vi "LCM_player.vi"() -> ()   [LabVIEW 2015]
uses:
  <vilib>/Utility/file.llb/Write To Spreadsheet File (DBL).vi
  G_LCM.vi
panel:
  out "size(s)":i32
  out "LCM error":errorcluster
  in  "long format":bool
  out "UDP Comm. Error 2":errorcluster
  out "Receive Buffer Size":u32
  out "recv data":string
  out "Array":string[](array[string])
  out "time":dbl
  out "log time":string
  in  "time-to-live":u16
  out "LCM":T1
  out "Wait for next data recv [sec]":dbl
  out "File Path":path
  in  "배속(0.1~10)":dbl=0.2 min=0.01 max=10.0 step=0.01
  out "t_old":i64
  out "idxtime":i64[](array[numeric])
  in  "Sequence Index Slider":i32(slide) scale=0.0..1387934.0
  out "idxsize":i32[](array[numeric])
  in  "Play/Pause":bool
  out "channel":string
  out "header":T2 {"magic" format="%08x"}
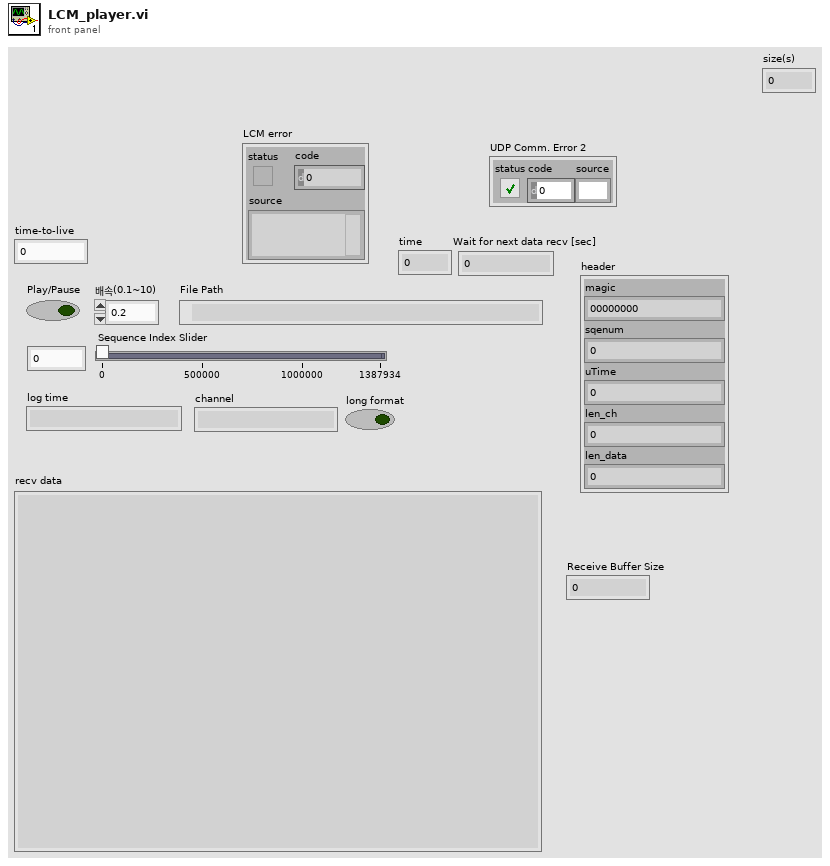
[diagram p1: front panel]
types:
  T1 = cluster{"connection ID":refnum<k16>, "net address":u32, "port":u16}
  T2 = cluster{"magic":i32, "sqenum":i64, "uTime":i64, "len_ch":i32, "len_data":i32}
  T3 = enum8{"Enabled", "Disabled", "Disabled and Grayed Out"}
  T4 = cluster{"magic":u32, "msg_seqno":u32, "msg_size":u32, "fragment_offset":u32, "fragment_no":u16, "fragments_in_msg":u16}
  T5 = cluster{"hash":i64, "sys time":i64, "time":dbl, "yaw_rate":dbl, "mdps torque":dbl, "mdps str_ang":dbl, "VS_CAN":dbl, "lat_accel":dbl, "mcp":dbl, "accel pedal value":dbl, "tps":dbl, "odometer":dbl, "battery voltage":dbl, "WHL_SPD_RR":dbl, "WHL_SPD_RL":dbl, "WHL_SPD_FR":dbl, "WHL_SPD_FL":dbl}
  T6 = cluster{"hash":dbl, "sys time":dbl, "time":dbl, "yaw_rate":dbl, "mdps torque":dbl, "mdps str_ang":dbl, "VS_CAN":dbl, "lat_accel":dbl, "mcp":dbl, "accel pedal value":dbl, "tps":dbl, "odometer":dbl, "battery voltage":dbl, "WHL_SPD_RR":dbl, "WHL_SPD_RL":dbl, "WHL_SPD_FR":dbl, "WHL_SPD_FL":dbl}
  T7 = cluster{"hash":i64, "sys time":i64, "time":dbl, "x":dbl, "y":dbl, "h":dbl, "numSV":i32, "postype":i32, "lag":i32, "hordev":dbl, "lat":dbl, "lon":dbl, "hgt":dbl, "map_idx":i32}
  T8 = cluster{"hash":dbl, "sys time":dbl, "time":dbl, "x":dbl, "y":dbl, "h":dbl, "numSV":dbl, "postype":dbl, "lag":dbl, "hordev":dbl, "lat":dbl, "lon":dbl, "hgt":dbl, "map_idx":dbl}
  T9 = cluster{"hash":i64, "sys time":i64, "time":dbl, "speed":dbl, "heading":dbl, "lat":dbl, "lon":dbl}
  T10 = cluster{"hash":dbl, "sys time":dbl, "time":dbl, "speed":dbl, "heading":dbl, "lat":dbl, "lon":dbl}
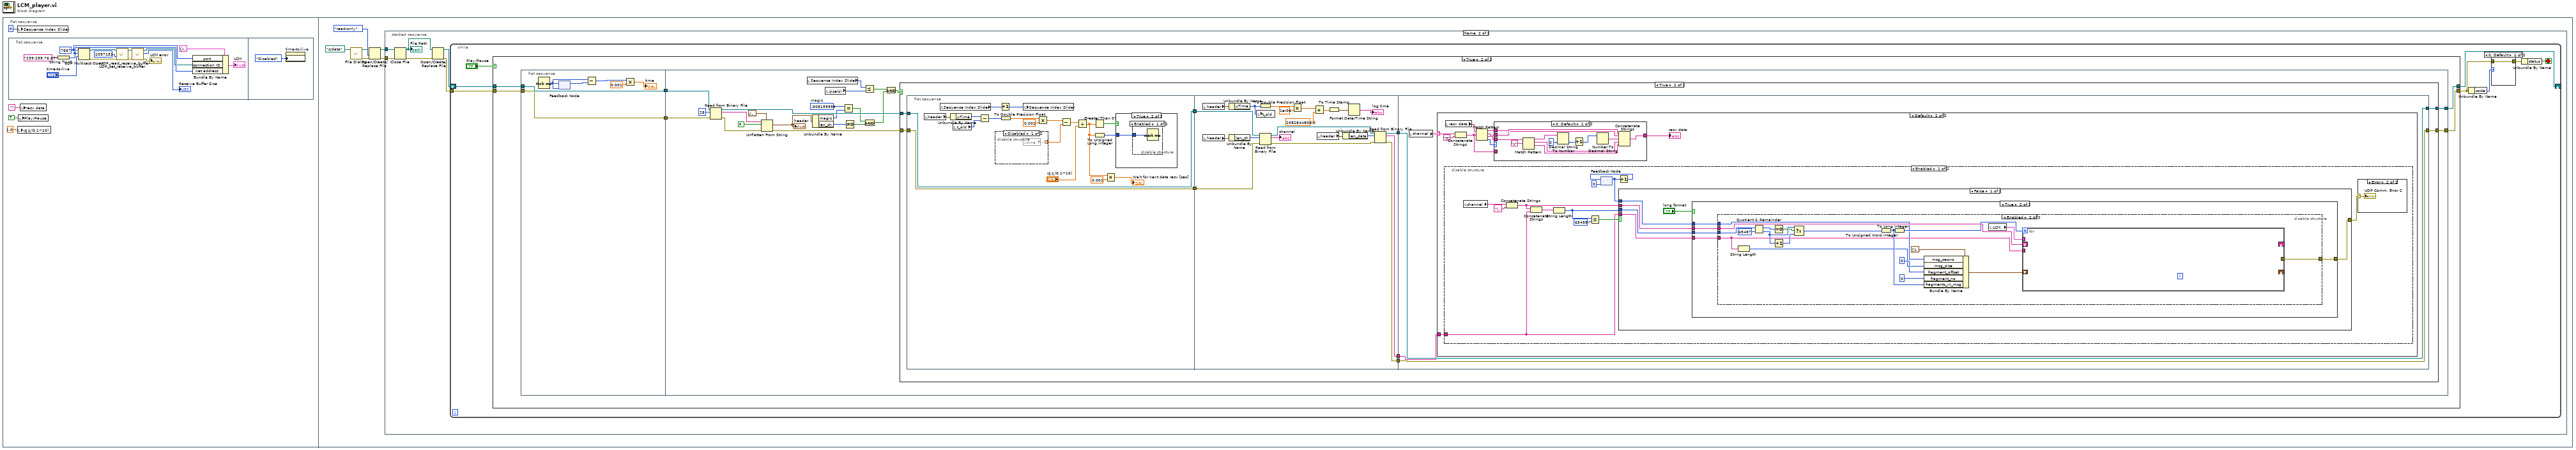
[diagram p0: block diagram]
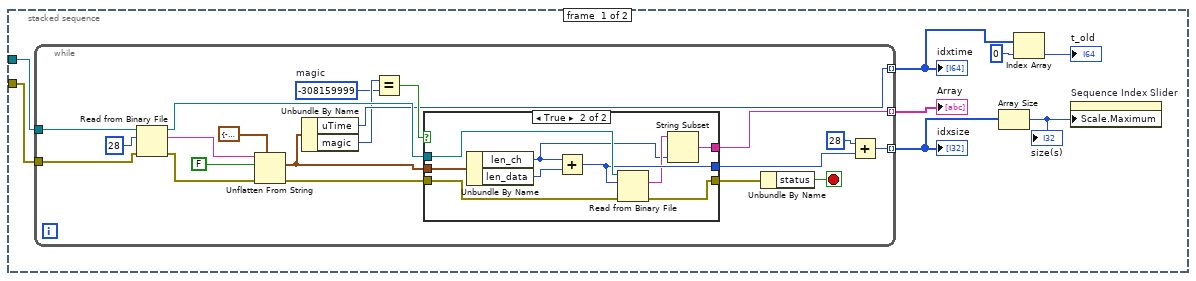
[diagram p2: hidden frame]
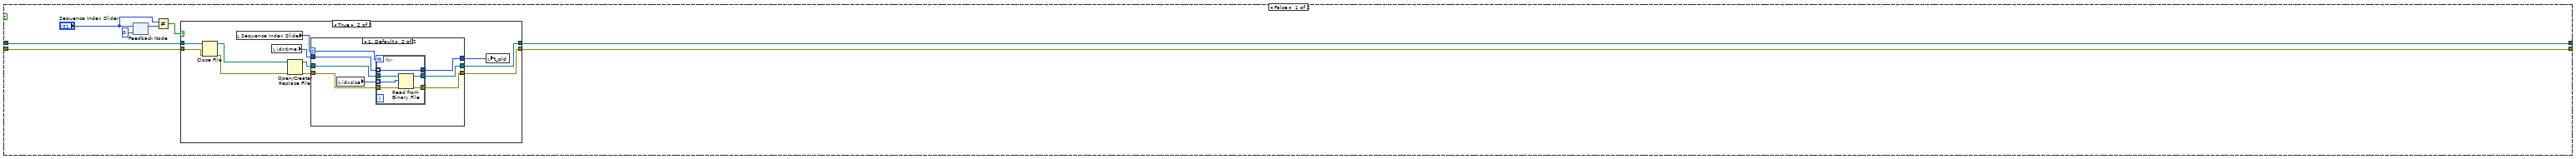
[diagram p5: hidden frame]
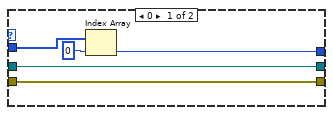
[diagram p7: hidden frame]
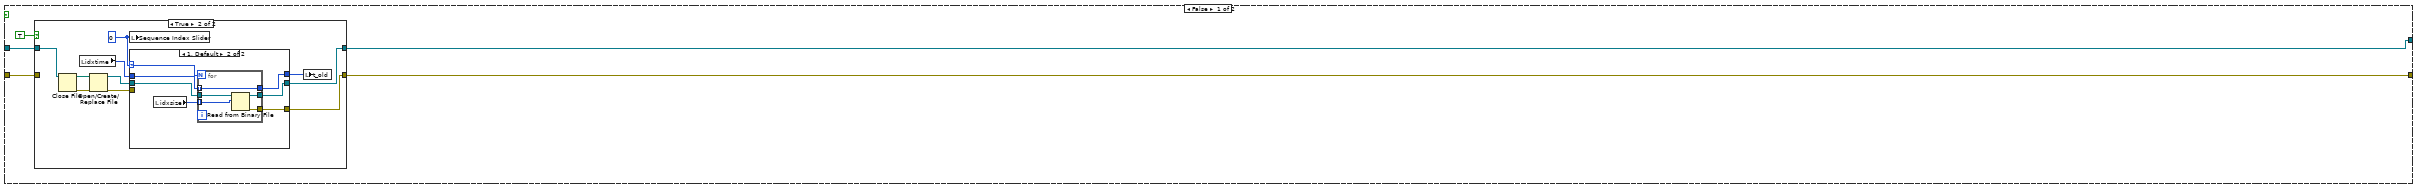
[diagram p8: hidden frame]
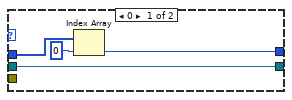
[diagram p10: hidden frame]
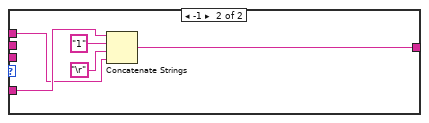
[diagram p15: hidden frame]
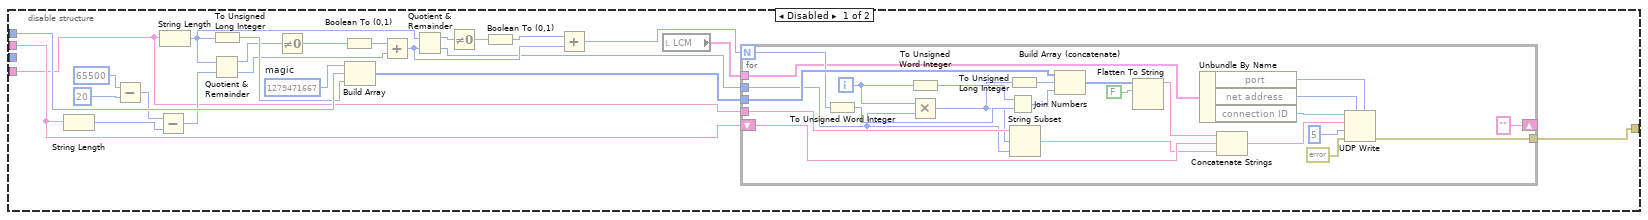
[diagram p17: hidden frame]
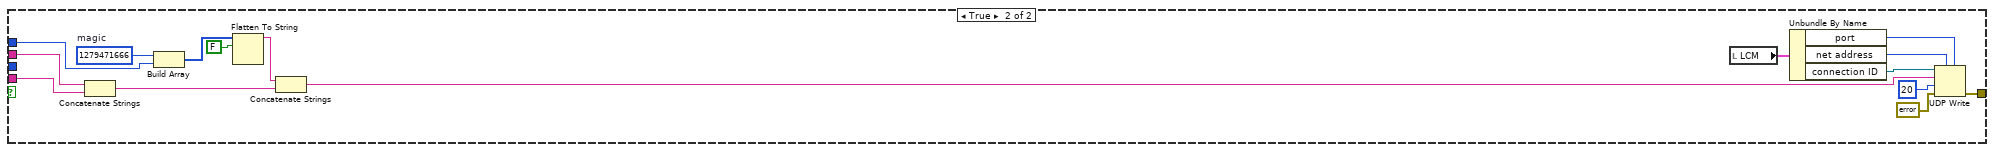
[diagram p18: hidden frame]
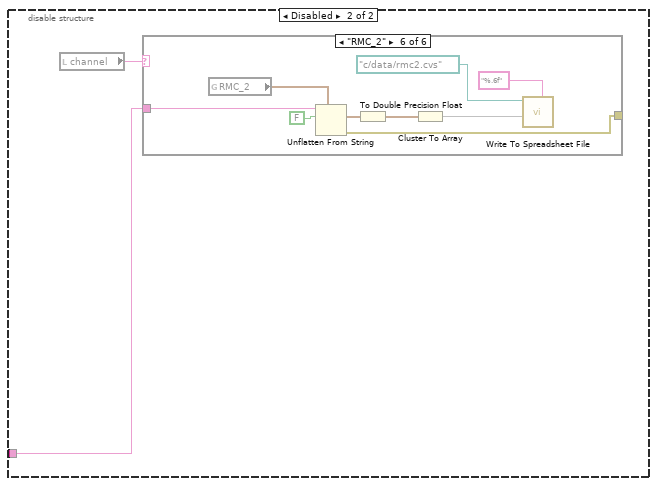
[diagram p20: hidden frame]
diagram:
  n1 = flat-sequence {
    frame #0 {
      n2 = flat-sequence {
        frame #0 {
          w13 = u16 7667 ("port")
          n3 = String To IP(1:"239.255.76.67" ("Multicast Address")) -> (0:w17:u32)
          n4 = UDP Multicast Open(9:"time-to-live", 10:w17, 11:w13) -> (0:w6:errorcluster, 3:w9:refnum<k16>)  [unwired: 2 in, 1 out]
          n5 = call "UDP_set_receive_buffer.vi"("error in (no error)"=w6, "Receive Buffer Size"=u32 2097152, "connection ID"=w9) -> ("error out"=w10:errorcluster, "connection ID out"=w8:refnum<k16>)  [unwired: 6 in]
          n6 = call "UDP_read_receive_buffer.vi"("error in (no error)"=w10, "connection ID"=w8) -> ("error out"=→"LCM error":errorcluster, "Receive Buffer Size"=→"Receive Buffer Size":u32, "connection ID out"=w7:refnum<k16>)  [unwired: 5 in]
          n7 = Bundle By Name(cluster=T1 {"connection ID"=refnum, "net address"=0, "port"=7667} ("LCM"), "port"=w13, "connection ID"=w7, "net address"=w17) -> (→"LCM":T1)
        }
        frame #1 {
          n8 = property on="time-to-live" class="DigNum (strict)"("DisabledEnum"=T3."Disabled" ("Disabled")) -> ()  [unwired: 2 in, 2 out]
        }
      }
      n9 = local write "Sequence Index Slider"(0 ("Slide")) -> ()
      n10 = local write "배속(0.1~10)"(1.0 ("배속(0.1~10)")) -> ()
      n11 = local write "Play/Pause"(TRUE ("play")) -> ()
      n12 = local write "recv data"("") -> ()
    }
    frame #1 {
      n13 = call "File Dialog"("start path"=path "c:/data") -> ("selected path"=w22:path, "error out"=w20:errorcluster)  [unwired: 11 in, 2 out]
      n14 = Open/Create/Replace File(file path (use dialog)=w22, error in=w20, access (0:read/write)=enum16{"read/write", "read-only", "write-only"}."read-only") -> (refnum out=w24:refnum<file>, error out=w25:errorcluster)  [unwired: 3 in, 1 out]
      n15 = stacked-sequence {
        tunnel: w24 -> [w33 w69]
        tunnel: w25 -> [w32 w68]
        frame #0 {
          n16 = while {
            tunnel: [w38] -> w31 mode=indexing
            tunnel: w33 -> [w51]
            tunnel: w32 -> [w39]
            tunnel: [w37] -> w29 mode=indexing
            tunnel: [w34] -> w26 mode=indexing
            stop <- w52 stop-if-true
            w35 = -308159999  # magic
            n17 = Read from Binary File(8:w39, 10:28 ("count (1)"), 11:w51) -> (0:w40:errorcluster, 2:w42:string, 3:w50:refnum<file>)  [unwired: 3 in, 1 out]
            n18 = Unflatten From String(type=T2 {"magic"=-308159999, "sqenum"=0, "uTime"=0, "len_ch"=0, "len_data"=0} ("header"), binary string=w42, data includes array or string size? (T)=FALSE, error in (no error)=w40) -> (value=w45:T2, error out=w48:errorcluster)  [unwired: 1 in, 1 out]
            n19 = Unbundle By Name(w45) -> ("uTime"=w37:i64, "magic"=w36:i32)
            n20 = Equal?(x=w36, y=w35) -> (x = y?=w49:bool)
            n21 = case shown="True" w49 {
              tunnel: w50 -> [_ w63]
              tunnel: [w54 w61] -> w53
              tunnel: w48 -> [w54 w62]
              tunnel: [_ w60] -> w47
              tunnel: w45 -> [_ w58]
              tunnel: [_ w55] -> w34
              frame False {
              }
              frame True {
                n22 = Unbundle By Name(w58) -> ("len_ch"=w56:i32, "len_data"=w59:i32)
                n23 = Add(x=w56, y=w59) -> (x+y=w60:i32)
                n24 = Read from Binary File(8:w62, 10:w60, 11:w63) -> (0:w61:errorcluster, 2:w57:string)  [unwired: 3 in, 2 out]
                n25 = String Subset(string=w57, length (rest)=w56) -> (substring=w55:string)  [unwired: 1 in]
              }
            }
            n26 = Unbundle By Name(w53) -> ("status"=w52:bool)
            n27 = Add(x=28 ("count (1)"), y=w47) -> (x+y=w38:i32)
          }
          "idxsize" <- w31
          "idxtime" <- w29
          "Array" <- w26
          n28 = Array Size(array=w31) -> (size(s)=w30:i32)
          "size(s)" <- w30
          n29 = Index Array(array=w29, index=0) -> (element=→"t_old":i64)
          n30 = property on="Sequence Index Slider" class="Slide (strict)"("Scale.Maximum"=w30) -> ()  [unwired: 2 in, 2 out]
        }
        frame #1 {
          n31 = Close File(refnum=w69, error in=w68) -> (path=w66:path, error out=w67:errorcluster)
          "File Path" <- w66
          n32 = Open/Create/Replace File(file path (use dialog)=w66, error in=w67) -> (refnum out=w65:refnum<file>, error out=w64:errorcluster)  [unwired: 4 in, 1 out]
          n33 = while {
            tunnel: w64 -> [w74]
            shift-right: [w73] -> _
            shift-left: w65 -> [w77]
            stop <- w76 stop-if-true
            n34 = case shown="True" "Play/Pause" {
              tunnel: w77 -> [w84 w124]
              tunnel: [w81 w123] -> w70
              tunnel: w74 -> [w83 w122]
              tunnel: [w82 w121] -> w73
              frame False {
                n35 = feedback-in #1("Sequence Index Slider") -> ()
                n36 = feedback #1(0 ("Slide")) -> (w79:i32)
                n37 = Not Equal?(x="Sequence Index Slider", y=w79) -> (x != y?=w85:bool)
                n38 = case shown="True" w85 {
                  tunnel: w84 -> [w88 w97]
                  tunnel: w83 -> [w87 w96]
                  tunnel: [w88 w93] -> w82
                  tunnel: [w87 w92] -> w81
                  frame False {
                  }
                  frame True {
                    n39 = Close File(refnum=w97, error in=w96) -> (path=w98:path, error out=w99:errorcluster)
                    n40 = local read "Sequence Index Slider"() -> (w89:i32)
                    n41 = local read "idxtime"() -> (w90:i64[])
                    n42 = Open/Create/Replace File(file path (use dialog)=w98, error in=w99) -> (refnum out=w95:refnum<file>, error out=w94:errorcluster)  [unwired: 4 in, 1 out]
                    n43 = case shown="1, Default" w89 {
                      selector: w89 -> [_ w105]
                      tunnel: w95 -> [w102 w112]
                      tunnel: w94 -> [w101 w111]
                      tunnel: [w102 w109] -> w93
                      tunnel: [w101 w108] -> w92
                      tunnel: [w103 w107] -> w91
                      tunnel: w90 -> [w104 w106]
                      frame 0 {
                        n44 = Index Array(array=w104, index=0) -> (element=w103:i64)
                      }
                      frame 1, Default {
                        n45 = local read "idxsize"() -> (w110:i32[])
                        n46 = for {
                          N: w105 -> [_]
                          tunnel: w112 -> [w118]
                          tunnel: w111 -> [w117]
                          tunnel: w110 -> [w116] mode=indexing
                          tunnel: [w115] -> w109
                          tunnel: [w114] -> w108
                          tunnel: [w113] -> w107
                          tunnel: w106 -> [w113] mode=indexing
                          n47 = Read from Binary File(8:w117, 10:w116, 11:w118) -> (0:w114:errorcluster, 3:w115:refnum<file>)  [unwired: 3 in, 2 out]
                        }
                      }
                    }
                    n48 = local write "t_old"(w91) -> ()
                  }
                }
              }
              frame True {
                n49 = flat-sequence {
                  tunnel: w122 -> [w130]
                  tunnel: w124 -> [w131]
                  tunnel: [w131] -> w120
                  tunnel: [w130] -> w119
                  tunnel: [w152] -> w123
                  tunnel: [w150] -> w121
                  tunnel: w120 -> [w153]
                  tunnel: w119 -> [w151]
                  frame #0 {
                    n50 = Tick Count (ms)() -> (millisecond timer value=w128:u32)
                    n51 = feedback-in #2(w128) -> ()
                    n52 = feedback #2(w128) -> (w129:u32)
                    n53 = Subtract(x=w128, y=w129) -> (x-y=w127:u32)
                    n54 = Multiply(x=w127, y=0.001) -> (x*y=→"time":dbl)
                  }
                  frame #1 {
                    w141 = -308159999  # magic
                    n55 = Read from Binary File(8:w151, 10:28 ("count (1)"), 11:w153) -> (0:w143:errorcluster, 2:w145:string, 3:w149:refnum<file>)  [unwired: 3 in, 1 out]
                    n56 = Unflatten From String(type=T2 {"magic"=-308159999, "sqenum"=0, "uTime"=0, "len_ch"=0, "len_data"=0} ("header"), binary string=w145, data includes array or string size? (T)=FALSE, error in (no error)=w143) -> (value=w142:T2, error out=w148:errorcluster)  [unwired: 1 in, 1 out]
                    "header" <- w142
                    n57 = local read "Sequence Index Slider"() -> (w136:i32)
                    n58 = Unbundle By Name(w142) -> ("magic"=w140:i32, "len_ch"=w139:i32)
                    n59 = local read "size(s)"() -> (w133:i32)
                    n60 = Equal?(x=w141, y=w140) -> (x = y?=w137:bool)
                    n61 = Not Equal To 0?(x=w139) -> (x != 0?=w138:bool)
                    n62 = Less Or Equal?(x=w136, y=w133) -> (x <= y?=w132:bool)
                    n63 = And(x=w137, y=w138) -> (x .and. y?=w134:bool)
                    n64 = And(x=w132, y=w134) -> (x .and. y?=w135:bool)
                    n65 = case shown="True" w135 {
                      tunnel: w149 -> [w158 w195]
                      tunnel: [w155 w191] -> w152
                      tunnel: w148 -> [w157 w192]
                      tunnel: [w156 w190] -> w150
                      frame False {
                        n66 = case shown="True" TRUE {
                          tunnel: w158 -> [w160 w168]
                          tunnel: w157 -> [w159 _]
                          tunnel: [w160 w165] -> w156
                          tunnel: [w159 w164] -> w155
                          frame False {
                          }
                          frame True {
                            w161 = 0 ("Sequence Index Slider")
                            n67 = Close File(refnum=w168) -> (path=w169:path, error out=w170:errorcluster)  [unwired: 1 in]
                            n68 = local read "idxtime"() -> (w162:i64[])
                            n69 = Open/Create/Replace File(file path (use dialog)=w169, error in=w170) -> (refnum out=w167:refnum<file>, error out=w166:errorcluster)  [unwired: 4 in, 1 out]
                            n70 = local write "Sequence Index Slider"(w161) -> ()
                            n71 = case shown="1, Default" w161 {
                              selector: w161 -> [_ w175]
                              tunnel: w167 -> [w172 w181]
                              tunnel: w166 -> [_ _]
                              tunnel: [w172 w179] -> w165
                              tunnel: [_ w178] -> w164
                              tunnel: [w173 w177] -> w163
                              tunnel: w162 -> [w174 w176]
                              frame 0 {
                                n72 = Index Array(array=w174, index=0) -> (element=w173:i64)
                              }
                              frame 1, Default {
                                n73 = local read "idxsize"() -> (w180:i32[])
                                n74 = for {
                                N: w175 -> [_]
                                tunnel: w181 -> [w186]
                                tunnel: w180 -> [w185] mode=indexing
                                tunnel: [w184] -> w179
                                tunnel: [w183] -> w178
                                tunnel: [w182] -> w177
                                tunnel: w176 -> [w182] mode=indexing
                                n75 = Read from Binary File(10:w185, 11:w186) -> (0:w183:errorcluster, 3:w184:refnum<file>)  [unwired: 4 in, 2 out]
                                }
                              }
                            }
                            n76 = local write "t_old"(w163) -> ()
                          }
                        }
                      }
                      frame True {
                        n77 = flat-sequence {
                          tunnel: [w214] -> w194
                          tunnel: [w208] -> w193
                          tunnel: w195 -> [w214]
                          tunnel: w192 -> [w208]
                          tunnel: w194 -> [w238]
                          tunnel: w193 -> [w226]
                          tunnel: [w220] -> w189
                          tunnel: [w225] -> w188
                          tunnel: [w221] -> w187
                          tunnel: [w241] -> w190
                          tunnel: [w242] -> w191
                          tunnel: w189 -> [w242]
                          tunnel: w188 -> [w241]
                          tunnel: w187 -> [w240]
                          frame #0 {
                            n78 = local read "header"() -> (w212:T2)
                            n79 = local read "Sequence Index Slider"() -> (w202:i32)
                            n80 = Unbundle By Name(w212) -> ("uTime"=w213:i64)
                            n81 = local read "t_old"() -> (w207:i64)
                            n82 = Subtract(x=w213, y=w207) -> (x-y=w211:i64)
                            n83 = disable-structure shown="Disabled" {
                              disable-tunnel: [w215 _] -> w198
                              frame Disabled {
                                n84 = local read "time"() -> (w215:dbl)
                              }
                              frame Enabled {
                              }
                            }
                            n85 = Increment(x=w202) -> (x+1=w203:i32)
                            n86 = To Double Precision Float(number=w211) -> (double precision float=w209:dbl)
                            n87 = local write "Sequence Index Slider"(w203) -> ()
                            n88 = Multiply(x=w209, y=0.001) -> (x*y=w197:dbl)
                            n89 = Subtract(x=w197, y=w198) -> (x-y=w196:dbl)
                            n90 = Divide(x=w196, y="배속(0.1~10)") -> (x/y=w200:dbl)
                            n91 = Greater Than 0?(x=w200) -> (x > 0?=w199:bool)
                            n92 = To Unsigned Long Integer(number=w200) -> (unsigned 32bit integer=w201:u32)
                            n93 = Multiply(x=w200, y=0.001) -> (x*y=→"Wait for next data recv [sec]":dbl)
                            n94 = case shown="True" w199 {
                              tunnel: w201 -> [_ w216]
                              frame False {
                              }
                              frame True {
                                n95 = disable-structure shown="Enabled" {
                                disable-tunnel: w216 -> [w217 _]
                                frame Enabled {
                                n96 = Wait (ms)(milliseconds to wait=w217) -> ()  [unwired: 1 out]
                                }
                                frame Disabled {
                                }
                                }
                              }
                            }
                          }
                          frame #1 {
                            n97 = local read "header"() -> (w229:T2)
                            n98 = local read "header"() -> (w237:T2)
                            n99 = Unbundle By Name(w229) -> ("uTime"=w224:i64)
                            n100 = Unbundle By Name(w237) -> ("len_ch"=w236:i32)
                            n101 = local write "t_old"(w224) -> ()
                            n102 = To Double Precision Float(number=w224) -> (double precision float=w233:dbl)
                            n103 = Read from Binary File(8:w226, 10:w236, 11:w238) -> (0:w219:errorcluster, 2:→"channel":string, 3:w227:refnum<file>)  [unwired: 3 in, 1 out]
                            n104 = Multiply(x=w233, y=1e-06) -> (x*y=w231:dbl)
                            n105 = Add(x=w231, y=2082844800.0 ("UTC+9h from 1970-01-01")) -> (x+y=w234:dbl)
                            n106 = local read "header"() -> (w228:T2)
                            n107 = To Time Stamp(1:w234) -> (0:w223:timestamp)
                            n108 = Unbundle By Name(w228) -> ("len_data"=w218:i32)
                            n109 = Format Date/Time String(seconds (now)=w223) -> (date/time string=→"log time":string)  [unwired: 2 in]
                            n110 = Read from Binary File(8:w219, 10:w218, 11:w227) -> (0:w220:errorcluster, 2:w221:string, 3:w225:refnum<file>)  [unwired: 3 in, 1 out]
                          }
                          frame #2 {
                            n111 = local read "channel"() -> (w239:string)
                            n112 = case shown="Default" w239 {
                              selector: w239 -> [_ w244]
                              tunnel: w240 -> [_ w243]
                              frame "" {
                              }
                              frame Default {
                                n113 = disable-structure shown="Enabled" {
                                disable-tunnel: w243 -> [w272 w400]
                                frame Enabled {
                                n114 = local read "channel"() -> (w277:string)
                                n115 = Concatenate Strings(w277, "\u0000" ("string")) -> (w271:string)
                                n116 = Concatenate Strings(w271, w272) -> (w273:string)
                                n117 = String Length(string=w273) -> (length=w270:i32)
                                n118 = Less Or Equal?(x=w270, y=65499 ("length (rest)")) -> (x <= y?=w274:bool)
                                n119 = feedback #3(u32 0) -> (w280:u32)
                                n120 = Increment(x=w280) -> (x+1=w281:u32)
                                n121 = feedback-in #3(w281) -> ()
                                n122 = case shown="False" w274 {
                                tunnel: w280 -> [w287 w396]
                                tunnel: [w284 w387] -> w278
                                tunnel: w272 -> [w285 w383]
                                tunnel: w271 -> [w286 w384]
                                tunnel: w270 -> [w282 _]
                                frame False {
                                n123 = case shown="True" "long format" {
                                tunnel: w287 -> [_ w292]
                                tunnel: w286 -> [_ w291]
                                tunnel: w285 -> [_ w290]
                                tunnel: [_ w289] -> w284
                                tunnel: w282 -> [_ w288]
                                frame False {
                                }
                                frame True {
                                n124 = disable-structure shown="Enabled" {
                                disable-tunnel: w292 -> [w315 w344]
                                disable-tunnel: w291 -> [w305 w346]
                                disable-tunnel: w290 -> [w304 w343]
                                disable-tunnel: [w294 w341] -> w289
                                disable-tunnel: w288 -> [_ w345]
                                frame Disabled {
                                w316 = u32 1279471667  # magic
                                n125 = String Length(string=w305) -> (length=w306:i32)
                                n126 = Subtract(x=65500 ("length (rest)"), y=20) -> (x-y=w309:i32)
                                n127 = Subtract(x=w309, y=w306) -> (x-y=w308:i32)
                                n128 = String Length(string=w304) -> (length=w303:i32)
                                n129 = To Unsigned Long Integer(number=w303) -> (unsigned 32bit integer=w311:u32)
                                n130 = Quotient & Remainder(x=w303, y=w308) -> (x-y*floor(x/y)=w299:i32, floor(x/y)=w297:i32)
                                n131 = Not Equal To 0?(x=w299) -> (x != 0?=w312:bool)
                                n132 = Boolean To (0,1)(Boolean=w312) -> (0, 1=w298:i16)
                                n133 = Build Array(w316, w315, w311) -> (w307:u32[])
                                n134 = Add(x=w298, y=w297) -> (x+y=w301:i32)
                                n135 = Quotient & Remainder(x=w303, y=w301) -> (x-y*floor(x/y)=w295:i32, floor(x/y)=w296:i32)
                                n136 = Not Equal To 0?(x=w295) -> (x != 0?=w310:bool)
                                n137 = Boolean To (0,1)(Boolean=w310) -> (0, 1=w302:i16)
                                n138 = Add(x=w302, y=w301) -> (x+y=w300:i32)
                                n139 = local read "LCM"() -> (w293:T1)
                                n140 = for {
                                N: w300 -> [w338]
                                tunnel: w296 -> [w326]
                                tunnel: w307 -> [w340]
                                shift-right: [""] -> _
                                shift-left: w305 -> [w329]
                                tunnel: w304 -> [w333]
                                tunnel: [w318] -> w294
                                tunnel: w293 -> [w317]
                                i -> [w325]
                                n141 = To Unsigned Word Integer(number=w338) -> (unsigned 16bit integer=w336:u16)
                                n142 = To Unsigned Word Integer(number=w325) -> (unsigned 16bit integer=w337:u16)
                                n143 = Multiply(x=w325, y=w326) -> (x*y=w327:i32)
                                n144 = Join Numbers(hi=w337, lo=w336) -> ((hi.lo)=w335:u32)
                                n145 = To Unsigned Long Integer(number=w327) -> (unsigned 32bit integer=w339:u32)
                                n146 = String Subset(string=w333, offset (0)=w327, length (rest)=w326) -> (substring=w328:string)
                                n147 = Build Array (concatenate)(w340, w339, w335) -> (w331:u32[])
                                n148 = Flatten To String(anything=w331, prepend array or string size? (T)=FALSE) -> (data string=w330:string)  [unwired: 2 in, 2 out]
                                n149 = Unbundle By Name(w317) -> ("port"=w322:u16, "net address"=w321:u32, "connection ID"=w320:refnum<k16>)
                                n150 = Concatenate Strings(w330, w329, w328) -> (w319:string)
                                n151 = UDP Write(address=w321, port or service name=w322, connection ID=w320, data in=w319, 8:errorcluster {"status"=FALSE, "code"=0, "source"=""} ("error in (no error)"), 9:5 ("timeout ms (25000)")) -> (error out=w318:errorcluster)  [unwired: 1 out]
                                }
                                }
                                frame Enabled {
                                n152 = String Length(string=w343) -> (length=w342:i32)
                                n153 = Quotient & Remainder(x=w345, y=65487) -> (x-y*floor(x/y)=w348:i32, floor(x/y)=w351:i32)
                                n154 = Equal To 0?(x=w348) -> (x = 0?=w349:bool)
                                n155 = Increment(x=w351) -> (x+1=w350:i32)
                                n156 = Select(t=w351, s=w349, f=w350) -> (s? t:f=w355:i32)
                                n157 = To Unsigned Word Integer(number=w355) -> (unsigned 16bit integer=w357:u16)
                                n158 = To Long Integer(number=w357) -> (32bit integer=w358:i32)
                                n159 = Bundle By Name(cluster=T4 {"magic"=1279471667, "msg_seqno"=1279471667, "msg_size"=1279471667, "fragment_offset"=1279471667, "fragment_no"=12339, "fragments_in_msg"=12339}, "msg_seqno"=w344, "msg_size"=w342, "fragment_offset"=u32 0, "fragment_no"=u16 0, "fragments_in_msg"=w357) -> (w359:T4)
                                n160 = local read "LCM"() -> (w347:T1)
                                n161 = for {
                                N: w358 -> [_]
                                shift-right: [""] -> _
                                shift-left: w346 -> [w376]
                                tunnel: w343 -> [w379]
                                tunnel: w347 -> [w369]
                                tunnel: [w367] -> w341
                                shift-right: [w364] -> _
                                shift-left: w359 -> [w363]
                                i -> [w366]
                                n162 = Unbundle By Name(w363) -> ("fragment_offset"=w362:u32)
                                n163 = String Length(string=w376) -> (length=w380:i32)
                                n164 = Flatten To String(anything=w363, prepend array or string size? (T)=FALSE) -> (data string=w374:string)  [unwired: 2 in, 2 out]
                                n165 = Subtract(x=65487 ("y"), y=w380) -> (x-y=w361:i32)
                                n166 = Add(x=w362, y=w361) -> (x+y=w360:u32)
                                n167 = String Subset(string=w379, offset (0)=w362, length (rest)=w361) -> (substring=w377:string)
                                n168 = Unbundle By Name(w369) -> ("port"=w370:u16, "net address"=w371:u32, "connection ID"=w372:refnum<k16>)
                                n169 = Concatenate Strings(w374, w376, w377) -> (w368:string)
                                n170 = Increment(x=w366) -> (x+1=w365:i32)
                                n171 = Bundle By Name(cluster=w363, "fragment_no"=w365, "fragment_offset"=w360) -> (w364:T4)
                                n172 = UDP Write(address=w371, port or service name=w370, connection ID=w372, data in=w368, 9:10 ("timeout ms (25000)")) -> (error out=w367:errorcluster)  [unwired: 1 in, 1 out]
                                }
                                }
                                }
                                }
                                }
                                }
                                frame True {
                                w393 = u32 1279471666  # magic
                                n173 = Concatenate Strings(w384, w383) -> (w382:string)
                                n174 = Build Array(w393, w396) -> (w394:u32[])
                                n175 = Flatten To String(anything=w394, prepend array or string size? (T)=FALSE) -> (data string=w386:string)  [unwired: 2 in, 2 out]
                                n176 = Concatenate Strings(w386, w382) -> (w385:string)
                                n177 = local read "LCM"() -> (w391:T1)
                                n178 = Unbundle By Name(w391) -> ("port"=w390:u16, "net address"=w389:u32, "connection ID"=w388:refnum<k16>)
                                n179 = UDP Write(address=w389, port or service name=w390, connection ID=w388, data in=w385, 8:errorcluster {"status"=FALSE, "code"=0, "source"=""} ("error in (no error)"), 9:20 ("timeout ms (25000)")) -> (error out=w387:errorcluster)  [unwired: 1 out]
                                }
                                }
                                n180 = case shown="Error" w278 {
                                selector: w278 -> [_ w398]
                                frame No Error {
                                }
                                frame Error {
                                "UDP Comm. Error 2" <- w398
                                }
                                }
                                }
                                frame Disabled {
                                n181 = local read "channel"() -> (w399:string)
                                n182 = case shown="\"RMC_2\"" w399 {
                                tunnel: w400 -> [_ w403 w412 w421 w430 w439]
                                tunnel: [_ w401 w410 w419 w428 w437] -> _
                                frame "False", Default {
                                }
                                frame "CAN_T" {
                                n183 = global read "G_LCM.vi" "CAN_T"() -> (w402:T5)
                                n184 = Unflatten From String(type=w402, binary string=w403, data includes array or string size? (T)=FALSE) -> (value=w408:T5, error out=w401:errorcluster)  [unwired: 2 in, 1 out]
                                n185 = To Double Precision Float(number=w408) -> (double precision float=w407:T6)
                                n186 = Cluster To Array(cluster=w407) -> (array=w406:dbl[])
                                n187 = call-poly <vilib>:"Write To Spreadsheet File.vi"("format (%.3f)"="%.6f", "1D data"=w406, "file path (dialog if empty)"=path "c:/data/can.cvs") -> ()  [unwired: 5 in, 1 out]
                                }
                                frame "GGA_1" {
                                n188 = global read "G_LCM.vi" "GGA_1"() -> (w411:T7)
                                n189 = Unflatten From String(type=w411, binary string=w412, data includes array or string size? (T)=FALSE) -> (value=w417:T7, error out=w410:errorcluster)  [unwired: 2 in, 1 out]
                                n190 = To Double Precision Float(number=w417) -> (double precision float=w416:T8)
                                n191 = Cluster To Array(cluster=w416) -> (array=w415:dbl[])
                                n192 = call-poly <vilib>:"Write To Spreadsheet File.vi"("format (%.3f)"="%.6f", "1D data"=w415, "file path (dialog if empty)"=path "c:/data/gga1.cvs") -> ()  [unwired: 5 in, 1 out]
                                }
                                frame "GGA_2" {
                                n193 = global read "G_LCM.vi" "GGA_2"() -> (w420:T7)
                                n194 = Unflatten From String(type=w420, binary string=w421, data includes array or string size? (T)=FALSE) -> (value=w426:T7, error out=w419:errorcluster)  [unwired: 2 in, 1 out]
                                n195 = To Double Precision Float(number=w426) -> (double precision float=w425:T8)
                                n196 = Cluster To Array(cluster=w425) -> (array=w424:dbl[])
                                n197 = call-poly <vilib>:"Write To Spreadsheet File.vi"("format (%.3f)"="%.6f", "1D data"=w424, "file path (dialog if empty)"=path "c:/data/gga2.cvs") -> ()  [unwired: 5 in, 1 out]
                                }
                                frame "RMC_1" {
                                n198 = global read "G_LCM.vi" "RMC_1"() -> (w429:T9)
                                n199 = Unflatten From String(type=w429, binary string=w430, data includes array or string size? (T)=FALSE) -> (value=w435:T9, error out=w428:errorcluster)  [unwired: 2 in, 1 out]
                                n200 = To Double Precision Float(number=w435) -> (double precision float=w434:T10)
                                n201 = Cluster To Array(cluster=w434) -> (array=w433:dbl[])
                                n202 = call-poly <vilib>:"Write To Spreadsheet File.vi"("format (%.3f)"="%.6f", "1D data"=w433, "file path (dialog if empty)"=path "c:/data/rmc1.cvs") -> ()  [unwired: 5 in, 1 out]
                                }
                                frame "RMC_2" {
                                n203 = global read "G_LCM.vi" "RMC_2"() -> (w438:T9)
                                n204 = Unflatten From String(type=w438, binary string=w439, data includes array or string size? (T)=FALSE) -> (value=w444:T9, error out=w437:errorcluster)  [unwired: 2 in, 1 out]
                                n205 = To Double Precision Float(number=w444) -> (double precision float=w443:T10)
                                n206 = Cluster To Array(cluster=w443) -> (array=w442:dbl[])
                                n207 = call-poly <vilib>:"Write To Spreadsheet File.vi"("format (%.3f)"="%.6f", "1D data"=w442, "file path (dialog if empty)"=path "c:/data/rmc2.cvs") -> ()  [unwired: 5 in, 1 out]
                                }
                                }
                                }
                                }
                                n208 = local read "recv data"() -> (w250:string)
                                n209 = Concatenate Strings(w244, "\t") -> (w246:string)
                                n210 = Match Pattern(string=w250, regular expression=w246) -> (before substring=w249:string, match substring=w248:string, after substring=w247:string, offset past match=w252:i32)  [unwired: 1 in]
                                n211 = case shown="0, Default" w252 {
                                tunnel: [w260 w269] -> w251
                                tunnel: w249 -> [w255 w265]
                                tunnel: w248 -> [w254 _]
                                tunnel: w247 -> [w253 _]
                                tunnel: w246 -> [_ w266]
                                frame 0, Default {
                                n212 = Match Pattern(string=w253, regular expression="\r") -> (before substring=w264:string, match substring=w262:string, after substring=w263:string)  [unwired: 1 in, 1 out]
                                n213 = Decimal String To Number(string=w264, default (0L)=u64 0 ("default (0 I32)")) -> (number=w257:u64)  [unwired: 1 in, 1 out]
                                n214 = Increment(x=w257) -> (x+1=w259:u64)
                                n215 = Number To Decimal String(number=w259) -> (decimal integer string=w258:string)  [unwired: 1 in]
                                n216 = Concatenate Strings(w255, w254, w258, w262, w263) -> (w260:string)
                                }
                                frame -1 {
                                n217 = Concatenate Strings(w266, "1", "\r", w265) -> (w269:string)
                                }
                                }
                                "recv data" <- w251
                              }
                            }
                          }
                        }
                      }
                    }
                  }
                }
              }
            }
            n218 = Unbundle By Name(w70) -> ("code"=w72:i32)
            n219 = case shown="0, Default" w72 {
              tunnel: [w78 _] -> w71
              tunnel: w70 -> [w78 _]
              frame 0, Default {
              }
              frame 4 {
              }
            }
            n220 = Unbundle By Name(w71) -> ("status"=w76:bool)
          }
        }
      }
    }
  }
